vi "P_regulering.vi"(9 "k_p":dbl, 10 "SP":dbl, 11 "DATA":dbl) -> (1 "p_p":dbl, 2 "e(t)":dbl, 3 "u_p":dbl)   [LabVIEW 2022 SP3]
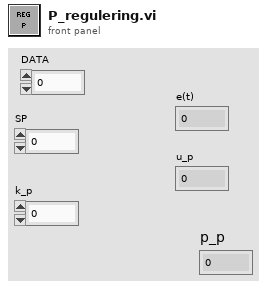
[diagram p1: front panel]
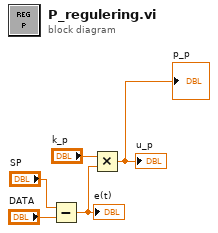
[diagram p0: block diagram]
diagram:
  n1 = Subtract(x="SP", y="DATA") -> (x-y=w4:dbl)
  "e(t)" <- w4
  n2 = Multiply(x="k_p", y=w4) -> (x*y=→"u_p" →"p_p":dbl)
